vi "CleanStartingEOL.vi"(2 "String":string) -> (16 "string":string)   [LabVIEW 2017, in "STOMP.lvclass"]
uses:
  STOMP.lvclass
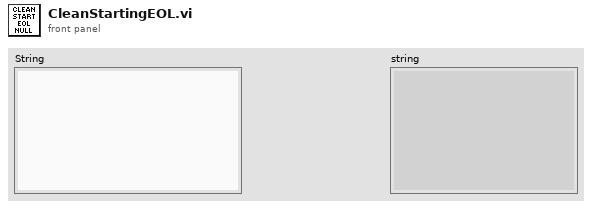
[diagram p1: front panel]
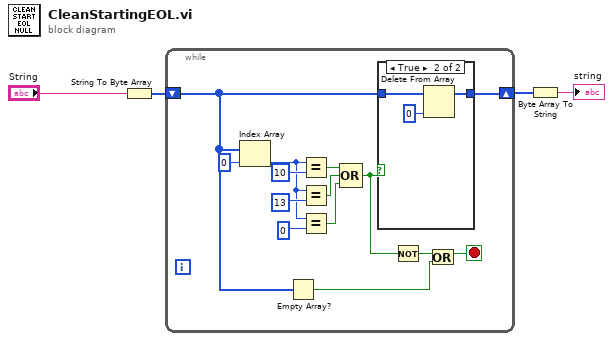
[diagram p0: block diagram]
diagram:
  n1 = String To Byte Array(string="String") -> (unsigned byte array=w4:u8[])
  n2 = while {
    shift-right: [w13] -> w3
    shift-left: w4 -> [w6]
    stop <- w7 stop-if-true
    n3 = Index Array(array=w6, index=0) -> (element=w9:u8)
    n4 = Empty Array?(array=w6) -> (empty?=w5:bool)
    n5 = Equal?(x=w9, y=u8 10) -> (x = y?=w14:bool)
    n6 = Equal?(x=w9, y=u8 13) -> (x = y?=w15:bool)
    n7 = Equal?(x=w9, y=u8 0) -> (x = y?=w8:bool)
    n8 = Compound Arithmetic op=OR(w14, w15, w8) -> (w12:bool)
    n9 = case shown="True" w12 {
      tunnel: w6 -> [w19 w22]
      tunnel: [w19 w20] -> w13
      frame False {
      }
      frame True {
        n10 = Delete From Array(array=w22, index=0) -> (array with subset deleted=w20:u8[])  [unwired: 1 in, 1 out]
      }
    }
    n11 = Not(x=w12) -> (.not. x?=w11:bool)
    n12 = Or(x=w11, y=w5) -> (x .or. y?=w7:bool)
  }
  n13 = Byte Array To String(unsigned byte array=w3) -> (string=→"string":string)
